vi "VI_Ppal.vi"() -> ()   [LabVIEW 2022 SP3]
panel:
  out "String":string
  out "?":bool
  in  "?":bool
  out "Tank":dbl(slide) scale=0.0..10.0
  in  "Válvula de salida":dbl(slide) scale=0.0..1.0 scale format="%#.1f"
  in  "Válvula de entrada":dbl(slide) scale=0.0..1.0 scale format="%#_1f"
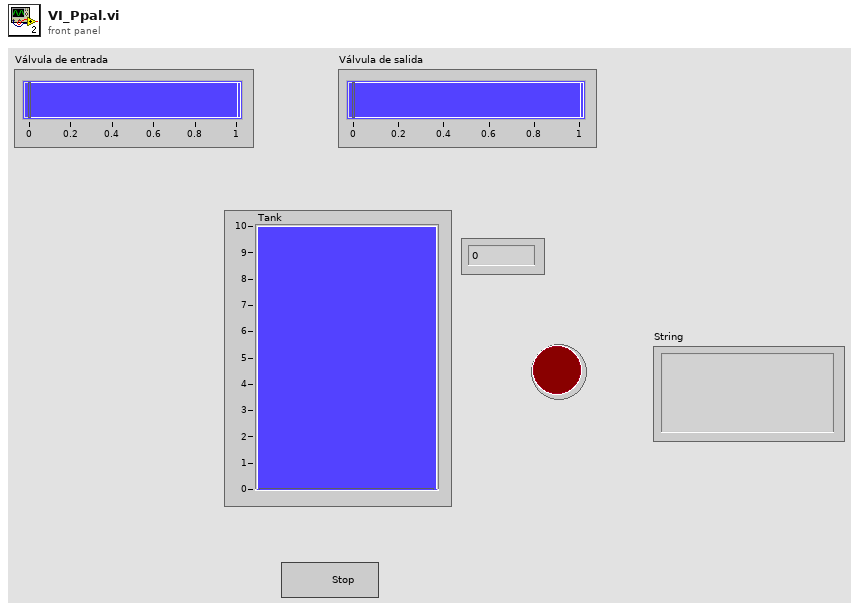
[diagram p1: front panel]
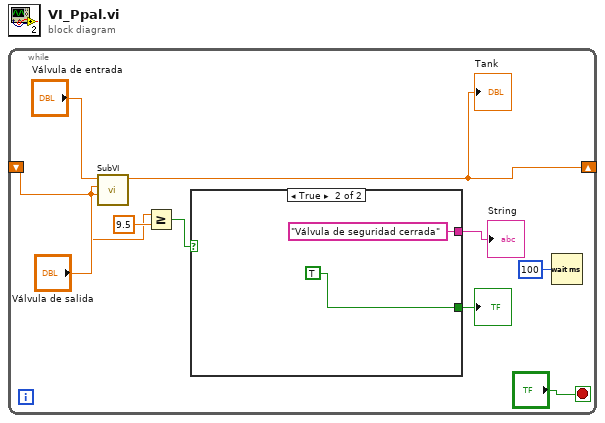
[diagram p0: block diagram]
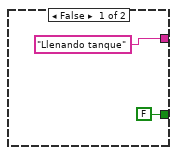
[diagram p2: hidden frame]
diagram:
  n1 = while {
    shift-right: [w5] -> _
    shift-left: _ -> [w2]
    stop <- "?" stop-if-true
    n2 = call "SubVI.vi"("ht"=w2, "uout"="Válvula de salida", "uin"="Válvula de entrada") -> ("Tank"=w5:dbl)  [unwired: 8 in]
    "Tank" <- w5
    n3 = Greater Or Equal?(x=w2, y=9.5) -> (x >= y?=w6:bool)
    n4 = case shown="True" w6 {
      tunnel: [FALSE TRUE] -> w3
      tunnel: ["Llenando tanque" "Válvula de seguridad cerrada"] -> w1
      frame False {
      }
      frame True {
      }
    }
    "?" <- w3
    "String" <- w1
    n5 = Wait (ms)(milliseconds to wait=u32 100) -> ()  [unwired: 1 out]
  }
